vi "Add Item to Tree.vi"(6 "Display Text Override":string, 8 "error in (no error)":errorcluster, 9 "Parent Tag":string, 10 "Data Item":refnum<class "Data Item.lvclass">, 11 "Tree Manager in":refnum<class "Tree Manager.lvclass">) -> (0 "error out":errorcluster, 2 "New Tag":string, 3 "Tree Manager out":refnum<class "Tree Manager.lvclass">)   [LabVIEW 2026, in "VILab.lvlib" / "Tree Manager.lvclass"]
uses:
  Tree Manager.lvclass
  Data Item/Data Item.lvclass
  Tree Manager.lvclass/Tree Manager.ctl
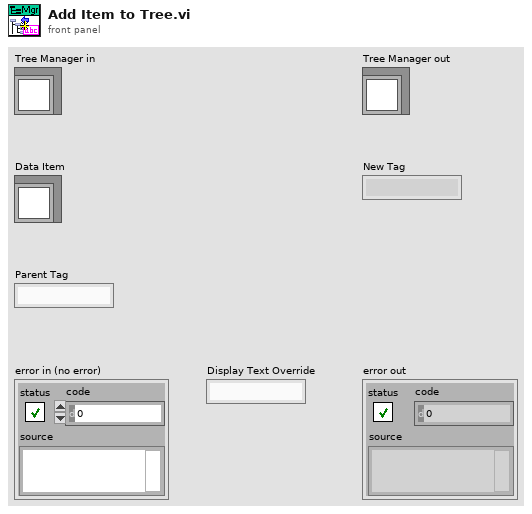
[diagram p1: front panel]
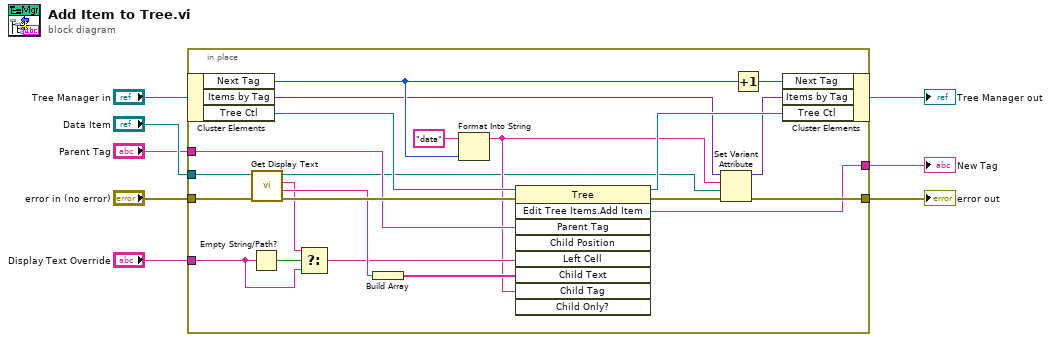
[diagram p0: block diagram]
diagram:
  n1 = in-place {
    in-place-border: "Data Item" -> [w26]
    in-place-border: "error in (no error)" -> [w30]
    in-place-border: "Parent Tag" -> [w24]
    in-place-border: [w16] -> w2
    in-place-border: "Display Text Override" -> [w10]
    in-place-border: [w27] -> w7
    n2 = in-place-cluster #1("Tree Manager in") -> ("Next Tag"=w18:u64, "Items by Tag"=w13:variant, "Tree Ctl"=w25:refnum<vi>)
    n3 = Empty String/Path?(string/path=w10) -> (empty?=w9:bool)
    n4 = call-dynamic "Get Display Text.vi"("error in (no error)"=w30, "Data Item in"=w26) -> ("error out"=w28:errorcluster, "Detail Text"=w23:string, "Display Name"=w12:string, "Data Item out"=w11:refnum<class "Data Item.lvclass">)  [unwired: 6 in]
    n5 = Select(t=w12, s=w9, f=w10) -> (s? t:f=w15:string)
    n6 = Build Array(w23) -> (w22:string[])
    n7 = Format Into String(initial string="data", w18) -> (resulting string=w14:string)  [unwired: 2 in, 1 out]
    n8 = invoke class="Tree" method="Edit Tree Items.Add Item"(reference=w25, error in=w28, "Parent Tag"=w24, "Left Cell"=w15, "Child Text"=w22, "Child Tag"=w14) -> (reference out=w21:refnum<vi>, error out=w29:errorcluster, "Edit Tree Items:Add Item"=w16:string)  [unwired: 3 in, 6 out]
    n9 = Set Variant Attribute(Variant=w13, name=w14, value=w11, error in=w29) -> (Variant out=w20:variant, error out=w27:errorcluster)  [unwired: 1 out]
    n10 = Increment(x=w18) -> (x+1=w19:u64)
    n11 = in-place-cluster #1("Next Tag"=w19, "Items by Tag"=w20, "Tree Ctl"=w21) -> (→"Tree Manager out":refnum<class "Tree Manager.lvclass">)
  }
  "error out" <- w7
  "New Tag" <- w2
